vi "database test.vi"() -> ()   [LabVIEW 2015]
uses:
  <vilib>/addons/database/Connection.llb/DB Tools Open Connec (String).vi
  <vilib>/addons/database/NI_Database_API.lvlib
panel:
  in  "SN":string="JJJJJ"
  in  "columns":string[](array[string])=["SN"]
  out "error out":errorcluster
  in  "ConnectionString":string="Driver=SQL Server;SERVER=PC-WEILY\\SQLEXPRESS;UID=sa;PWD=weilynare;DATABASE=PACK_SQLDATA;"
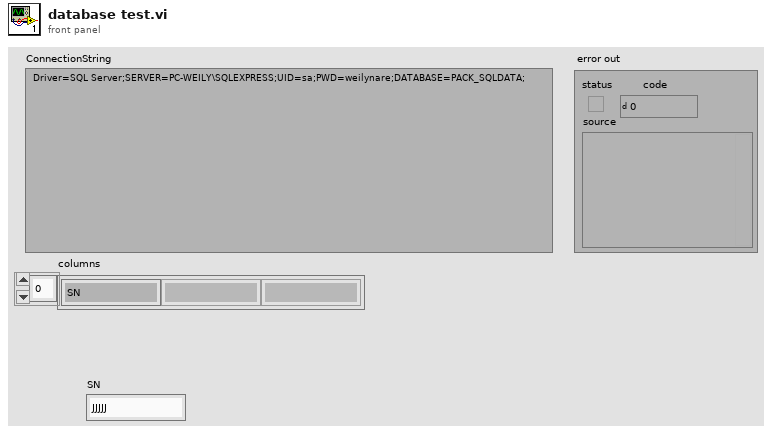
[diagram p1: front panel]
types:
  T1 = typedef "NI_Database_API.lvlib/Conn ObjectReference.ctl" = refnum<k1>
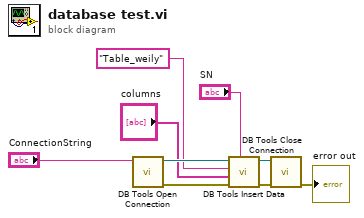
[diagram p0: block diagram]
diagram:
  n1 = call-poly <vilib>:"DB Tools Open Connection.vi"("connection information"="ConnectionString") -> ("error out"=w8:errorcluster, "connection reference"=w7:T1)  [unwired: 7 in]
  n2 = call <vilib>:"DB Tools Insert Data.vi"("data"="SN", "error in (no error)"=w8, "columns"="columns", "table"="Table_weily", "connection reference"=w7) -> ("error out"=w5:errorcluster, "connection reference out"=w4:T1)  [unwired: 5 in]
  n3 = call <vilib>:"DB Tools Close Connection.vi"("error in (no error)"=w5, "connection reference"=w4) -> ("error out"=→"error out":errorcluster)  [unwired: 5 in]
